vi "ReplaceSubVINode.vi"(5 "Old File Name":string, 7 "New File Name":string, 8 "error in (no error)":errorcluster, 11 "VI Refnum In":refnum<vi>) -> (0 "error out":errorcluster, 3 "VI Refnum Out":refnum<vi>, 4 "Replaced":bool)   [LabVIEW 2024]
uses:
  <vilib>/Utility/traverseref.llb/TRef TravTarget.ctl
  <vilib>/Utility/traverseref.llb/VI Scripting - Traverse.lvlib
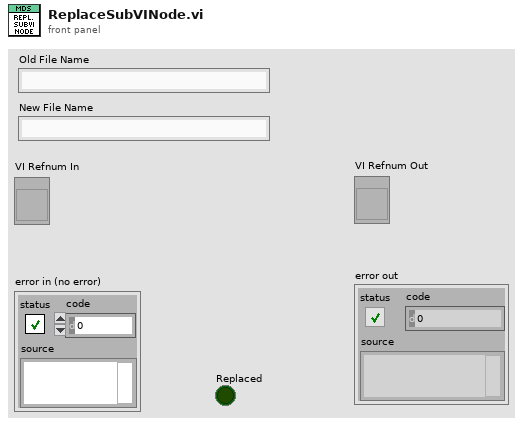
[diagram p1: front panel]
types:
  T1 = typedef "TRef TravTarget.ctl" = enum16{"FP", "BD", "Other"}
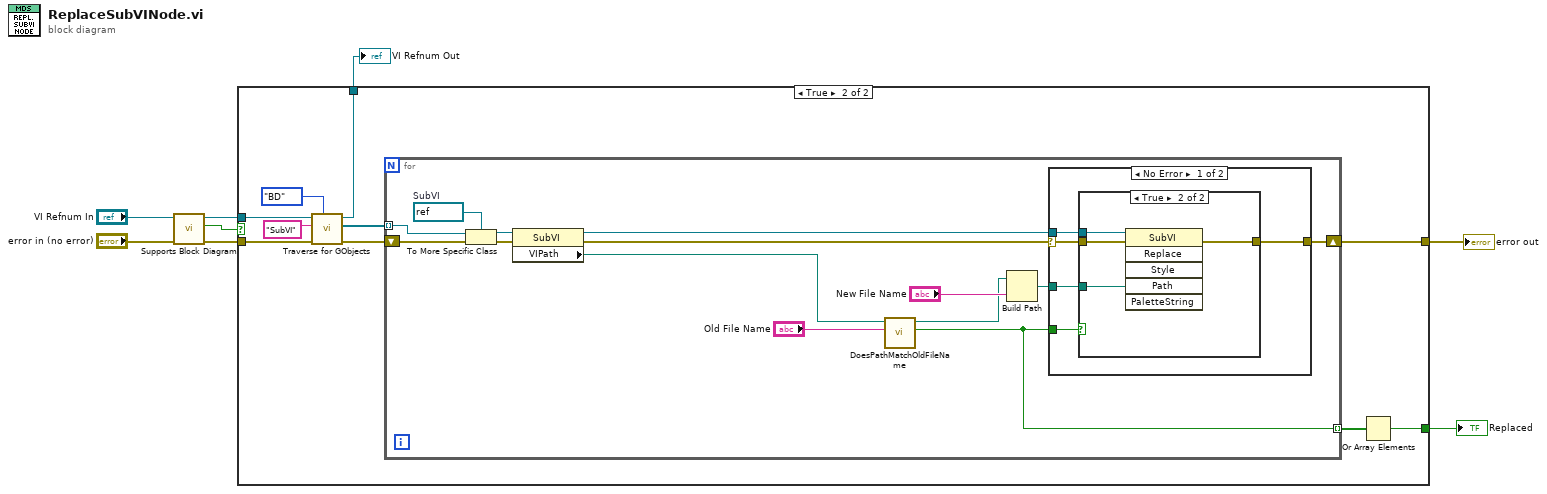
[diagram p0: block diagram]
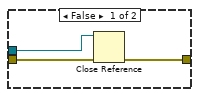
[diagram p3: hidden frame]
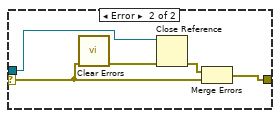
[diagram p4: hidden frame]
diagram:
  n1 = call "Supports Block Diagram.vi"("error in (no error)"="error in (no error)", "vi in"="VI Refnum In") -> ("error out"=w3:errorcluster, "has block diagram"=w1:bool, "vi out"=w2:refnum<vi>)  [unwired: 7 in]
  n2 = case shown="True" w1 {
    tunnel: w2 -> [w9 w16]
    tunnel: w3 -> [w10 w15]
    tunnel: [_ w11] -> w8
    tunnel: [w10 w14] -> w7
    tunnel: [w9 w13] -> w6
    frame False {
    }
    frame True {
      n3 = call <vilib>:"Traverse for GObjects.vi"("Traverse Target"=TRef_TravTarget."BD", "error in (no error)"=w15, "Class Name"="SubVI", "VI Refnum"=w16) -> ("error out"=w19:errorcluster, "References"=w20:refnum<vi>[], "dup VI Refnum"=w13:refnum<vi>)  [unwired: 4 in, 1 out]
      n4 = for {
        shift-right: [w29] -> w14
        shift-left: w19 -> [w30]
        tunnel: w20 -> [w31] mode=indexing
        tunnel: [w25] -> w12 mode=indexing
        w32 = refnum<vi> refnum  # SubVI
        n5 = To More Specific Class(target class=w32, reference=w31, error in=w30) -> (specific class reference=w33:refnum<vi>, error out=w34:errorcluster)
        n6 = property class="SubVI"(reference=w33, error in=w34) -> (reference out=w22:refnum<vi>, error out=w23:errorcluster, "VIPath"=w21:path)
        n7 = call "DoesPathMatchOldFileName.vi"("Old File Name"="Old File Name", "File Path"=w21) -> ("Match Found"=w25:bool, "Parent Directory"=w24:path)  [unwired: 8 in]
        n8 = Build Path(base path=w24, name or relative path="New File Name") -> (appended path=w28:path)
        n9 = case shown="No Error" w23 {
          selector: w23 -> [w35 w49]
          tunnel: w28 -> [w39 _]
          tunnel: w25 -> [w38 _]
          tunnel: [w37 w47] -> w29
          tunnel: w22 -> [w36 w50]
          frame No Error {
            n10 = case shown="True" w38 {
              tunnel: w39 -> [_ w46]
              tunnel: w35 -> [w42 w45]
              tunnel: [w41 w43] -> w37
              tunnel: w36 -> [w40 w44]
              frame False {
                n11 = Close Reference(reference=w40, error in (no error)=w42) -> (error out=w41:errorcluster)
              }
              frame True {
                n12 = invoke class="SubVI" method="Replace"(reference=w44, error in=w45, "Path"=w46) -> (error out=w43:errorcluster)  [unwired: 3 in, 5 out]
              }
            }
          }
          frame Error {
            n13 = call <vilib>:"Clear Errors.vi"("error in (no error)"=w49) -> ("error out"=w51:errorcluster)  [unwired: 5 in, 1 out]
            n14 = Close Reference(reference=w50, error in (no error)=w51) -> (error out=w48:errorcluster)
            n15 = Merge Errors(w48, w49) -> (w47:errorcluster)
          }
        }
      }
      n16 = Or Array Elements(Boolean array=w12) -> (logical OR=w11:bool)
    }
  }
  "error out" <- w7
  "Replaced" <- w8
  "VI Refnum Out" <- w6
